vi "Draw box(origin based).vi"(0 "Image":T2, 1 "Height factor":sgl=1.0, 2 "Width factor":dbl=2.0 format="%#_13g", 3 "Fixed overlay details":T1={"Overlay coordinates"=[], "Config coordinates"=[], "Inspection mode?"=TRUE}, 5 "Size bias factor":sgl, 7 "Color Box":u32(colorbox), 9 "Origin":cluster{"X":sgl, "Y":sgl}, 11 "error in (no error)":errorcluster, 12 "Drawing Mode (Frame)":u32(ring) items=["Frame", "Fill"], 13 "Group name":string, 14 "Start index":i32) -> (4 "Image Out":T2, 6 "Right adjacent origin":cluster{"X":sgl, "Y":sgl}, 8 "Bounding rectangle array":cluster{"X":dbl, "Y":dbl}[](array[cluster]), 10 "Overlay coordinates out":cluster{"X":dbl, "Y":dbl}[](array[cluster]), 15 "error out":errorcluster)   [LabVIEW 2019]
uses:
  <vilib>/vision/Image Controls.llb/IMAQ Image.ctl
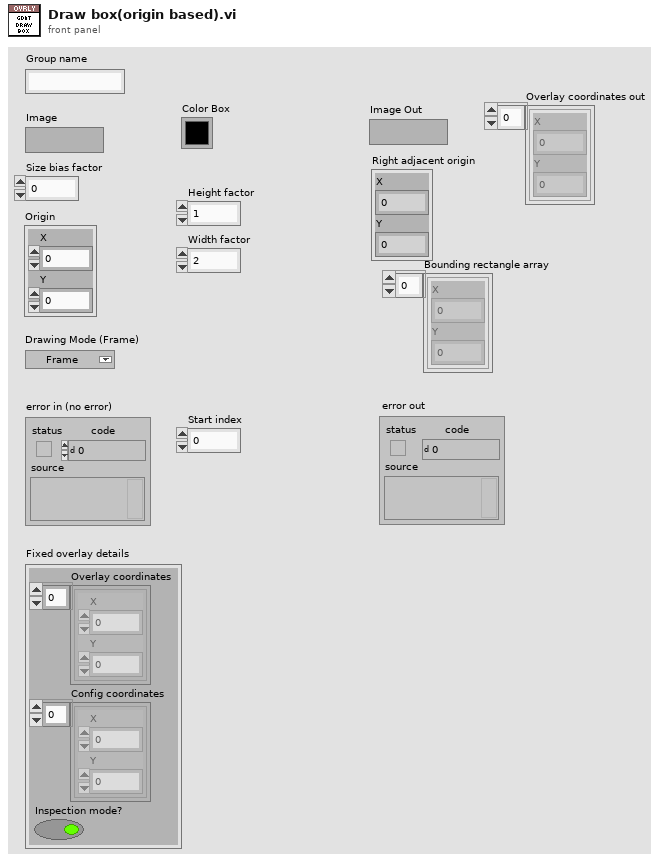
[diagram p1: front panel]
types:
  T1 = cluster{"Overlay coordinates":cluster{"X":dbl, "Y":dbl}[], "Config coordinates":cluster{"X":dbl, "Y":dbl}[], "Inspection mode?":bool}
  T2 = typedef "IMAQ Image.ctl" = refnum<image>
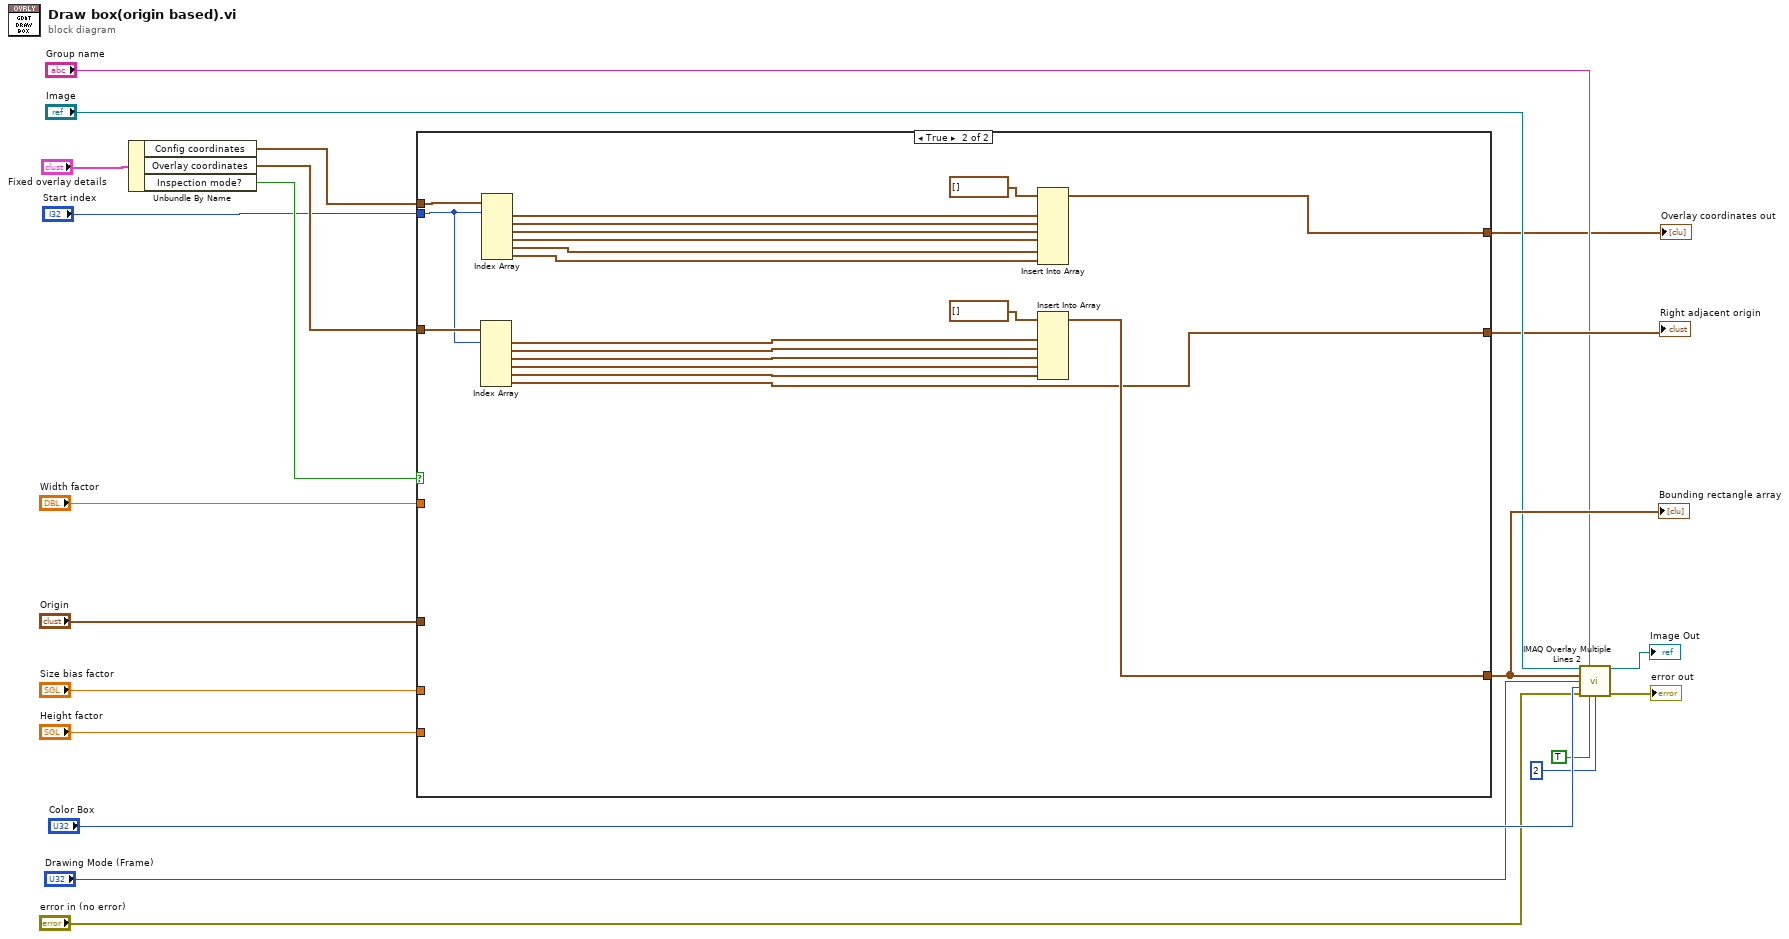
[diagram p0: block diagram]
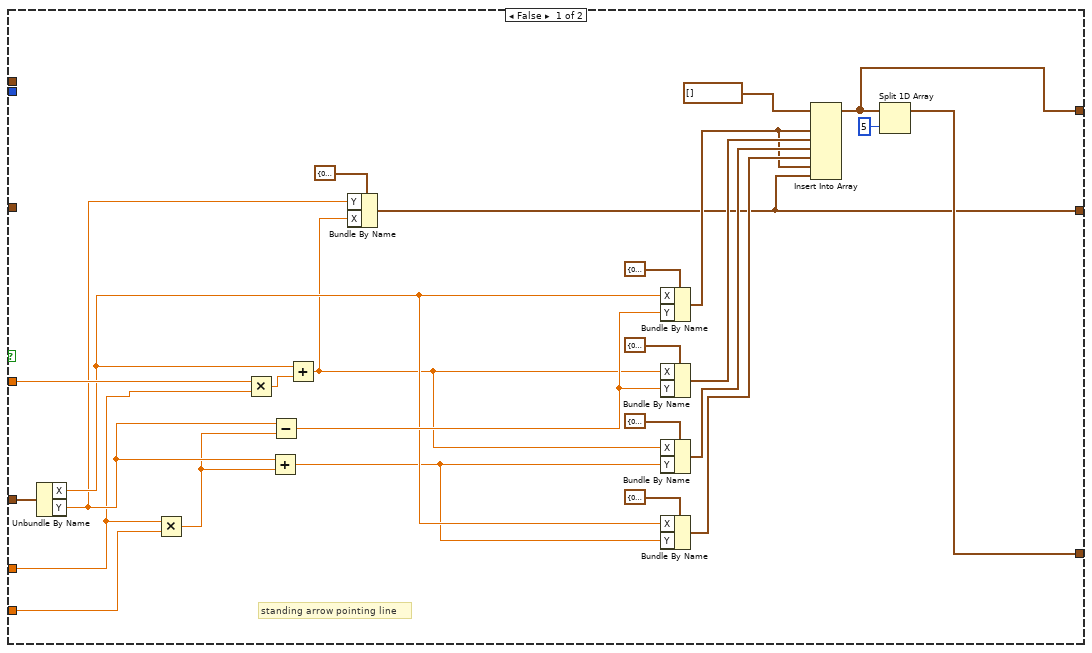
[diagram p2: hidden frame]
diagram:
  n1 = Unbundle By Name("Fixed overlay details") -> ("Config coordinates"=w4:cluster{"X":dbl, "Y":dbl}[], "Overlay coordinates"=w3:cluster{"X":dbl, "Y":dbl}[], "Inspection mode?"=w2:bool)
  n2 = case shown="True" w2 {
    tunnel: "Width factor" -> [w46 _]
    tunnel: "Origin" -> [w38 _]
    tunnel: [w24 w59] -> w19
    tunnel: "Size bias factor" -> [w33 _]
    tunnel: "Height factor" -> [w32 _]
    tunnel: [w22 w48] -> w10
    tunnel: [w23 w49] -> w6
    tunnel: w4 -> [_ w51]
    tunnel: w3 -> [_ w50]
    tunnel: "Start index" -> [_ w47]
    frame False {
      # "standing arrow pointing line"
      n3 = Unbundle By Name(w38) -> ("X"=w39:sgl, "Y"=w34:sgl)
      n4 = Multiply(x=w33, y=w32) -> (x*y=w31:sgl)
      n5 = Multiply(x=w46, y=w33) -> (x*y=w45:dbl)
      n6 = Add(x=w34, y=w31) -> (x+y=w37:sgl)
      n7 = Subtract(x=w34, y=w31) -> (x-y=w40:sgl)
      n8 = Add(x=w39, y=w45) -> (x+y=w35:dbl)
      n9 = Bundle By Name(cluster=cluster{"X":sgl, "Y":sgl} {"X"=0.0, "Y"=0.0} ("Origin 2"), "Y"=w34, "X"=w35) -> (w22:cluster{"X":sgl, "Y":sgl})
      n10 = Bundle By Name(cluster=cluster{"X":dbl, "Y":dbl} {"X"=0.0, "Y"=0.0} ("Point Coordinates"), "X"=w39, "Y"=w40) -> (w26:cluster{"X":dbl, "Y":dbl})
      n11 = Bundle By Name(cluster=cluster{"X":dbl, "Y":dbl} {"X"=0.0, "Y"=0.0} ("Point Coordinates"), "X"=w35, "Y"=w40) -> (w29:cluster{"X":dbl, "Y":dbl})
      n12 = Bundle By Name(cluster=cluster{"X":dbl, "Y":dbl} {"X"=0.0, "Y"=0.0} ("Point Coordinates"), "X"=w35, "Y"=w37) -> (w28:cluster{"X":dbl, "Y":dbl})
      n13 = Bundle By Name(cluster=cluster{"X":dbl, "Y":dbl} {"X"=0.0, "Y"=0.0} ("Point Coordinates"), "X"=w39, "Y"=w37) -> (w27:cluster{"X":dbl, "Y":dbl})
      n14 = Insert Into Array(array=cluster{"X":dbl, "Y":dbl}[] [], new element #1=w26, new element #2=w29, new element #3=w28, new element #4=w27, new element #5=w26, new element #6=w22) -> (w23:cluster{"X":dbl, "Y":dbl}[])  [unwired: 1 in]
      n15 = Split 1D Array(array=w23, index=5) -> (first subarray=w24:cluster{"X":dbl, "Y":dbl}[])  [unwired: 1 out]
    }
    frame True {
      n16 = Index Array(array=w50, index #1=w47) -> (element #1=w65:cluster{"X":dbl, "Y":dbl}, element #2=w64:cluster{"X":dbl, "Y":dbl}, element #3=w63:cluster{"X":dbl, "Y":dbl}, element #4=w62:cluster{"X":dbl, "Y":dbl}, element #5=w60:cluster{"X":dbl, "Y":dbl}, element #6=w48:cluster{"X":dbl, "Y":dbl})  [unwired: 5 in]
      n17 = Index Array(array=w51, index #1=w47) -> (element #1=w57:cluster{"X":dbl, "Y":dbl}, element #2=w56:cluster{"X":dbl, "Y":dbl}, element #3=w55:cluster{"X":dbl, "Y":dbl}, element #4=w54:cluster{"X":dbl, "Y":dbl}, element #5=w53:cluster{"X":dbl, "Y":dbl}, element #6=w52:cluster{"X":dbl, "Y":dbl})  [unwired: 5 in]
      n18 = Insert Into Array(array=cluster{"X":dbl, "Y":dbl}[] [], new element #1=w57, new element #2=w56, new element #3=w55, new element #4=w54, new element #5=w53, new element #6=w52) -> (w49:cluster{"X":dbl, "Y":dbl}[])  [unwired: 1 in]
      n19 = Insert Into Array(array=cluster{"X":dbl, "Y":dbl}[] [], new element #1=w65, new element #2=w64, new element #3=w63, new element #4=w62, new element #5=w60) -> (w59:cluster{"X":dbl, "Y":dbl}[])  [unwired: 1 in]
    }
  }
  "Right adjacent origin" <- w10
  "Bounding rectangle array" <- w19
  "Overlay coordinates out" <- w6
  n20 = call "IMAQ Overlay Multiple Lines 2"("Image"="Image", "Group"="Group name", "Line End Points"=w19, "Drawing Mode (Frame)"="Drawing Mode (Frame)", "Color"="Color Box", "error in (no error)"="error in (no error)", "Maintain Width?"=TRUE, "Width"=u32 2) -> ("Image Out"=→"Image Out":T2, "error out"=→"error out":errorcluster)  [unwired: 6 in]
